vi "HRM-GUI-main.vi"(8 "error in (no error)":errorcluster, 11 "init cluster":T1) -> (0 "error out":errorcluster)   [LabVIEW 2020]
uses:
  init/HRM-init-cluster.ctl
  init/HRM-init-user_events.ctl
panel:
  in  "Additional Signal to remove [s]":i32
  in  "samples [s]":i32=10
  in  "stop":bool
  out "Filtered data":waveform(dbl)(graph)
  out "Raw collected data":waveform(dbl)(graph)
  out "Heart Rate":dbl format="%.2p"
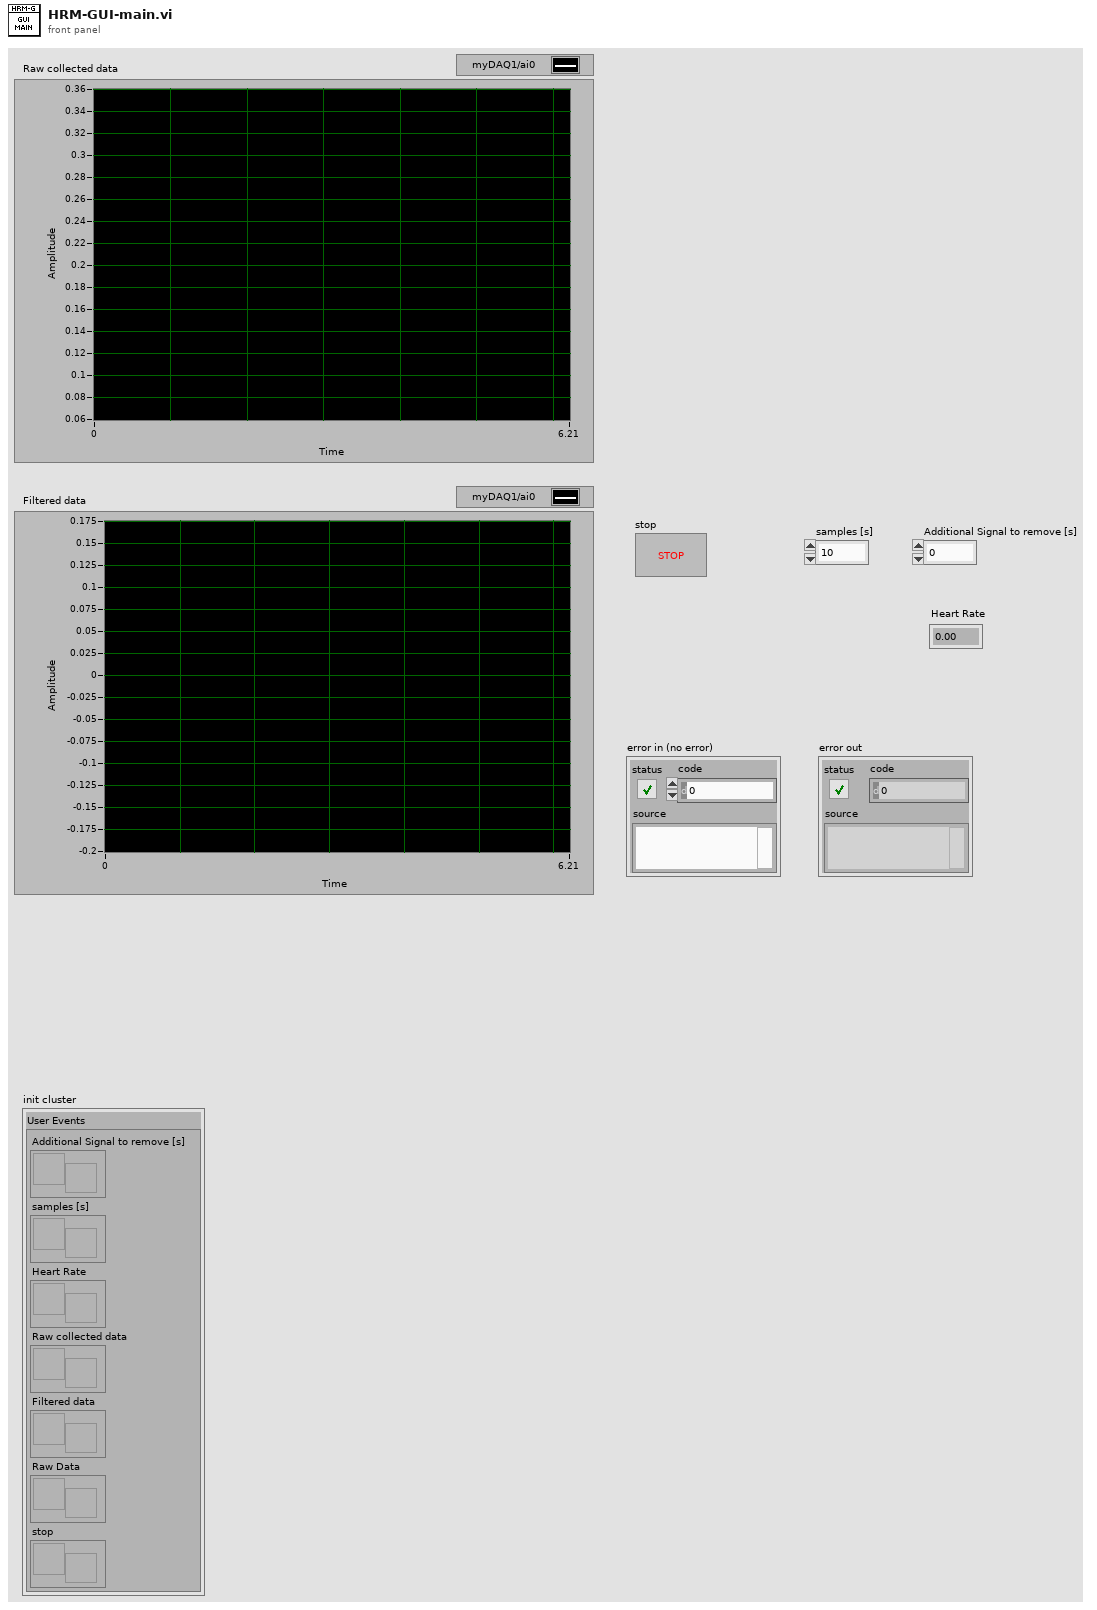
[diagram p1: front panel]
types:
  T1 = typedef "HRM-init-cluster.ctl" = cluster{"User Events":T2}
  T2 = typedef "HRM-init-user_events.ctl" = cluster{"Additional Signal to remove [s]":refnum<user-event>, "samples [s]":refnum<user-event>, "Heart Rate":refnum<user-event>, "Raw collected data":refnum<user-event>, "Filtered data":refnum<user-event>, "Raw Data":refnum<user-event>, "stop":refnum<user-event>}
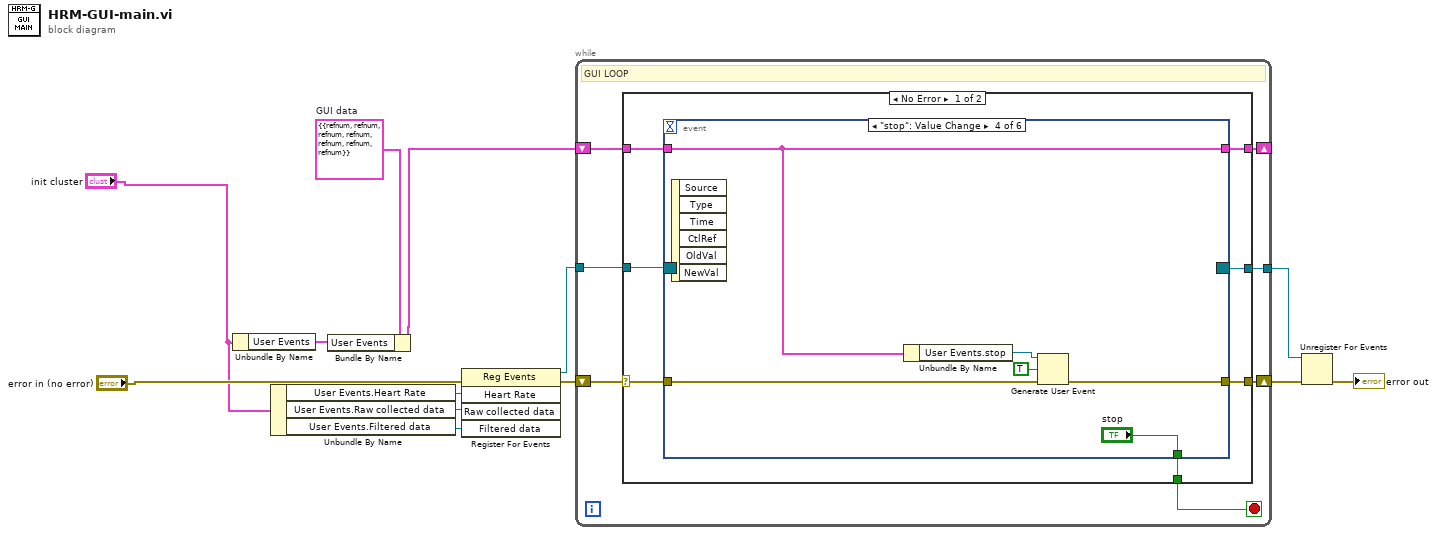
[diagram p0: block diagram]
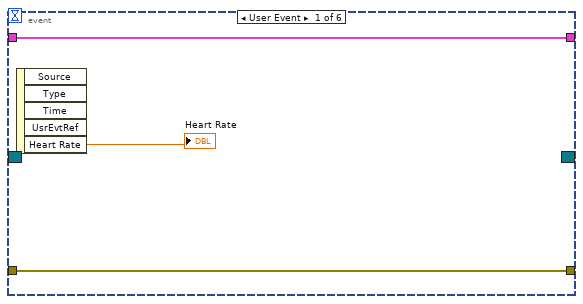
[diagram p2: hidden frame]
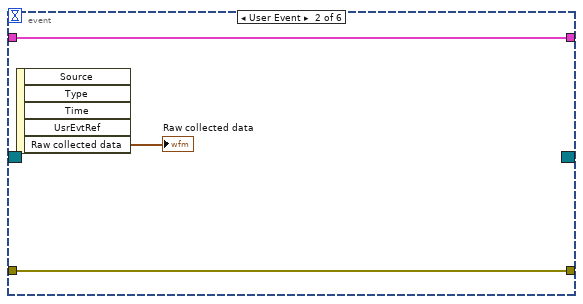
[diagram p3: hidden frame]
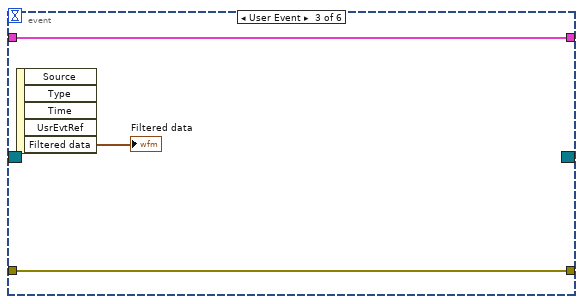
[diagram p4: hidden frame]
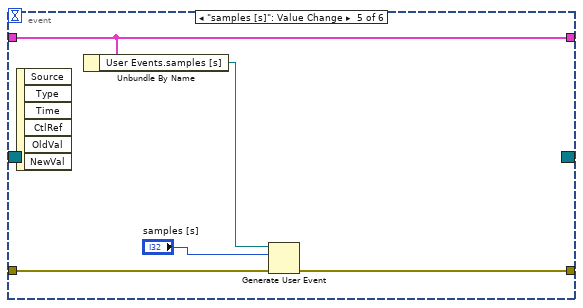
[diagram p5: hidden frame]
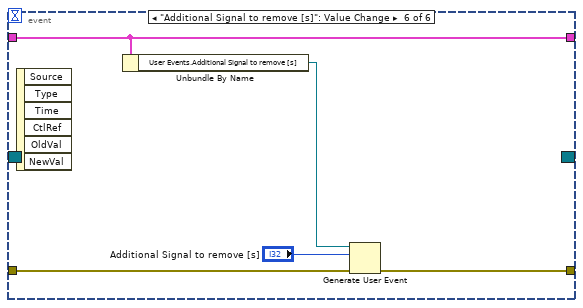
[diagram p6: hidden frame]
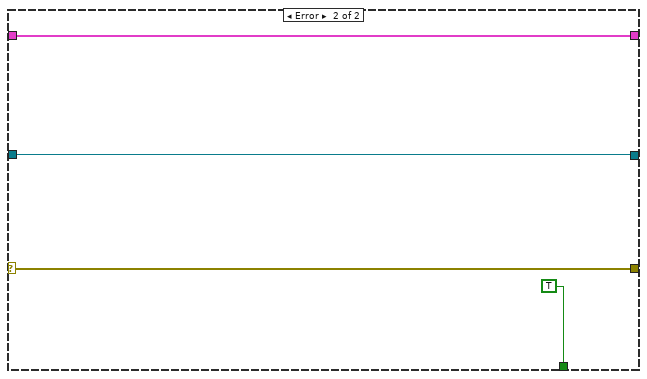
[diagram p7: hidden frame]
diagram:
  w8 = cluster{"User Events":T2} {"User Events"={"Additional Signal to remove [s]"=refnum, "samples [s]"=refnum, "Heart Rate"=refnum, "Raw collected data"=refnum, "Filtered data"=refnum, "Raw Data"=refnum, "stop"=refnum}}  # GUI data
  n1 = Unbundle By Name("init cluster") -> ("User Events"=w6:T2)
  n2 = Unbundle By Name("init cluster") -> ("User Events.Heart Rate"=w13:refnum<user-event>, "User Events.Raw collected data"=w5:refnum<user-event>, "User Events.Filtered data"=w4:refnum<user-event>)
  n3 = Bundle By Name(cluster=w8, "User Events"=w6) -> (w7:cluster{"User Events":T2})
  n4 = register-events(error in="error in (no error)", w13, w5, w4) -> (reference out=w9:refnum<event-registration>, error out=w10:errorcluster)  [unwired: 1 in]
  n5 = while {
    shift-right: [w19] -> w12
    shift-left: w10 -> [w20]
    tunnel: w9 -> [w17]
    tunnel: [w16] -> w11
    shift-right: [w15] -> _
    shift-left: w7 -> [w14]
    stop <- w18 stop-if-true
    # "GUI LOOP"
    n6 = case shown="No Error" w20 {
      selector: w20 -> [w27 w56]
      tunnel: [w22 w56] -> w19
      tunnel: [w21 TRUE] -> w18
      tunnel: w17 -> [w26 w54]
      tunnel: [w25 w54] -> w16
      tunnel: [w24 w53] -> w15
      tunnel: w14 -> [w23 w53]
      frame No Error {
        n7 = event shown="[3] \"stop\": Value Change" {
          selector: w26 -> [_ _ _ _ _ _]
          dyn-events: [_ _ _ _ _ _] -> w25
          timeout: _ -> [_ _ _ _ _ _]
          tunnel: w27 -> [w29 w33 w35 w41 w45 w50]
          tunnel: [w28 w31 w34 w39 w47 w52] -> w24
          tunnel: w23 -> [w28 w31 w34 w39 w47 w52]
          tunnel: [w29 w33 w35 w40 w44 w49] -> w22
          tunnel: [_ _ _ "stop" _ _] -> w21
          event User Event {
            n8 = event-data() -> ("Heart Rate"=→"Heart Rate":dbl)  [unwired: 1 in, 4 out]
          }
          event User Event {
            n9 = event-data() -> ("Raw collected data"=→"Raw collected data":waveform(dbl))  [unwired: 1 in, 4 out]
          }
          event User Event {
            n10 = event-data() -> ("Filtered data"=→"Filtered data":waveform(dbl))  [unwired: 1 in, 4 out]
          }
          event "stop": Value Change {
            n11 = event-data() -> ()  [unwired: 1 in, 6 out]
            n12 = Unbundle By Name(w39) -> ("User Events.stop"=w38:refnum<user-event>)
            n13 = Generate User Event(user event=w38, event data cluster=TRUE ("event data"), error in=w41) -> (error out=w40:errorcluster)  [unwired: 1 in, 1 out]
          }
          event "samples [s]": Value Change {
            n14 = event-data() -> ()  [unwired: 1 in, 6 out]
            n15 = Unbundle By Name(w47) -> ("User Events.samples [s]"=w46:refnum<user-event>)
            n16 = Generate User Event(user event=w46, event data cluster="samples [s]", error in=w45) -> (error out=w44:errorcluster)  [unwired: 1 in, 1 out]
          }
          event "Additional Signal to remove [s]": Value Change {
            n17 = event-data() -> ()  [unwired: 1 in, 6 out]
            n18 = Unbundle By Name(w52) -> ("User Events.Additional Signal to remove [s]"=w51:refnum<user-event>)
            n19 = Generate User Event(user event=w51, event data cluster="Additional Signal to remove [s]", error in=w50) -> (error out=w49:errorcluster)  [unwired: 1 in, 1 out]
          }
        }
      }
      frame Error {
      }
    }
  }
  n20 = Unregister For Events(event registration refnum=w11, error in=w12) -> (error out=→"error out":errorcluster)
